vi "MPM_Get_Sweep_Speed.vi"(8 "error in (no error)":errorcluster, 11 ".NET Reference in":refnum<k24>) -> (0 "error out":errorcluster, 2 "speed":dbl, 3 "Reference out":refnum<k24>)   [LabVIEW 2017]
uses:
  C:/Users/Ssantec_Test/Documents/Instrument_DLL_Sample_Labview_20250826_Ver1.5.0_x64/DLL/InstrumentDLL.dll
  DLL/InstrumentDLL.dll
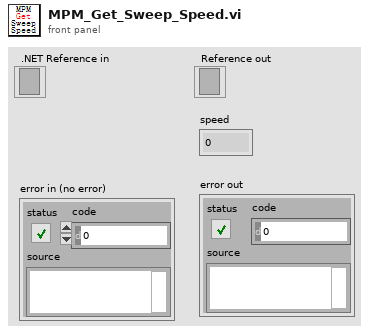
[diagram p1: front panel]
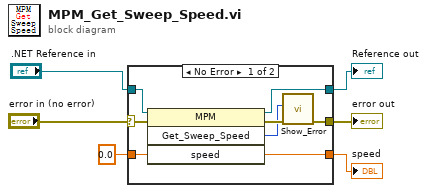
[diagram p0: block diagram]
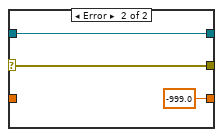
[diagram p2: hidden frame]
diagram:
  n1 = case shown="No Error" "error in (no error)" {
    selector: "error in (no error)" -> [w10 w15]
    tunnel: [w14 -999.0 ("speed")] -> w6
    tunnel: ".NET Reference in" -> [w13 w16]
    tunnel: [w12 w16] -> w4
    tunnel: 0.0 ("speed") -> [w11 _]
    tunnel: [w7 w15] -> w1
    frame No Error {
      n2 = invoke class="MPM" method="Get_Sweep_Speed"(reference=w13, error in=w10, "speed"=w11) -> (reference out=w12:refnum<k24>, error out=w9:errorcluster, "Get_Sweep_Speed"=w8:i32, "speed"=w14:dbl)  [unwired: 1 in]
      n3 = call "Show_Error.vi"("error in (no error)"=w9, "Error"=w8) -> ("error out"=w7:errorcluster)  [unwired: 9 in]
    }
    frame Error {
    }
  }
  "speed" <- w6
  "Reference out" <- w4
  "error out" <- w1
